vi "DestroyStandardEvents.vi"(8 "error in":errorcluster, 11 "standard events":T1) -> (0 "error out":errorcluster)   [LabVIEW 2025, in "CEF.lvlib" / "CEF_Node.lvclass"]
doc: "Copyright 2017 National Instruments Corporation\n\nLicensed under the Apache License, Version 2.0 (the \"License\"); you may not use this file except in compliance with the License. You may obtain a copy of the License at http://www.apache.org/licenses/LICENSE-2.0\nUnless required by applicable law or agreed to in writing, software distributed under the License is distributed on an \"AS IS\" BASIS, WITHOUT WARRANTIES OR CONDITIONS OF ANY KIND, either express or implied. See the License for the specific language governing permissions and limitations under the License."
uses:
  CEF_Node.lvclass
  StandardEvents.ctl
  UserEventRef.ctl
  Controls/EventCluster.ctl
  NodeChangeEvent.ctl
  NodeRef.ctl
  CacheState.ctl
  RefreshUIEvent.ctl
  StopEvent.ctl
  CEF_Node.lvclass/CEF_Node.ctl
  CEF.lvlib
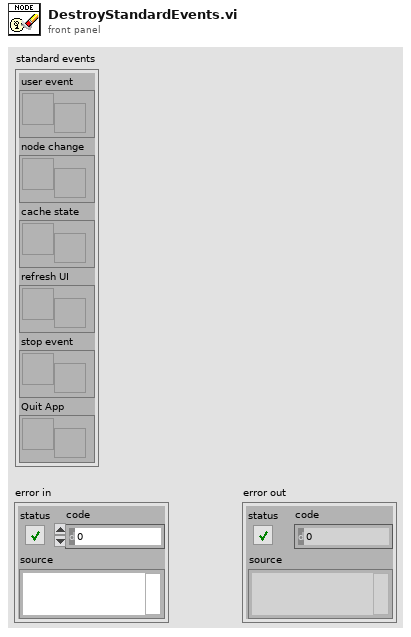
[diagram p1: front panel]
types:
  T1 = typedef "CEF.lvlib/CEF_Node.lvclass/StandardEvents.ctl" = cluster{"user event":T2, "node change":T3, "cache state":T4, "refresh UI":T5, "stop event":T6, "Quit App":refnum<user-event>}
  T2 = typedef "CEF.lvlib/CEF_Node.lvclass/UserEventRef.ctl" = refnum<user-event>
  T3 = typedef "CEF.lvlib/CEF_Node.lvclass/NodeChangeEvent.ctl" = refnum<user-event>
  T4 = typedef "CEF.lvlib/CEF_Node.lvclass/CacheState.ctl" = refnum<user-event>
  T5 = typedef "CEF.lvlib/CEF_Node.lvclass/RefreshUIEvent.ctl" = refnum<user-event>
  T6 = typedef "CEF.lvlib/CEF_Node.lvclass/StopEvent.ctl" = refnum<user-event>
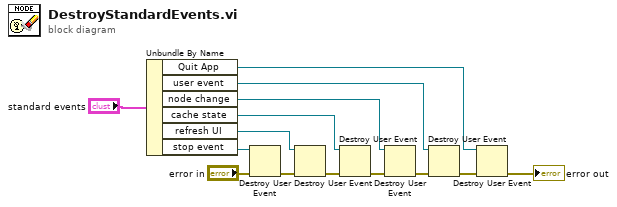
[diagram p0: block diagram]
diagram:
  n1 = Unbundle By Name("standard events") -> ("Quit App"=w1:refnum<user-event>, "user event"=w4:T2, "node change"=w5:T3, "cache state"=w6:T4, "refresh UI"=w7:T5, "stop event"=w8:T6)
  n2 = Destroy User Event(user event=w8, error in="error in") -> (error out=w12:errorcluster)
  n3 = Destroy User Event(user event=w7, error in=w12) -> (error out=w11:errorcluster)
  n4 = Destroy User Event(user event=w6, error in=w11) -> (error out=w10:errorcluster)
  n5 = Destroy User Event(user event=w5, error in=w10) -> (error out=w9:errorcluster)
  n6 = Destroy User Event(user event=w4, error in=w9) -> (error out=w3:errorcluster)
  n7 = Destroy User Event(user event=w1, error in=w3) -> (error out=→"error out":errorcluster)
